vi "test_ads_surface_vapor.vi"() -> ()   [LabVIEW 2017]
doc: "Minimal example that demonstrates functions implemented in the SorpPropLib for adsorption working pairs based on the surface approach and using the vapor pressure as additional property."
panel:
  out "Der. of loading wrt. pressure":cluster{dbl[], dbl[]}[](graph)=[{[100.0, 101.0, 102.0, 103.0, 104.0, 105.0, 106.0, 107.0, 108.0, 109.0], [0.00023285248517238496, 0.0002319852444530851, 0.00023112973054732367, 0.00023028567222781486, 0.00022945280709583772, 0.00022863088121227149, 0.0002278196487473965, 0.000227018871648338, 0.00022622831932311063, 0.00022544776834028737]}, {[100.0, 101.0, 102.0, 103.0, 104.0, 105.0, 106.0, 107.0, 108.0, 109.0], [0.00023285248517238496, 0.0002319852444530851, 0.00023112973054732367, 0.00023028567222781486, 0.00022945280709583772, 0.00022863088121227149, 0.0002278196487473965, 0.000227018871648338, 0.00022622831932311063, 0.00022544776834028737]}]
  out "Der. of loading wrt. temperature":cluster{dbl[], dbl[]}[](graph)=[{[100.0, 101.0, 102.0, 103.0, 104.0, 105.0, 106.0, 107.0, 108.0, 109.0], [-0.0013688715249931432, -0.00137741100365092, -0.001385918834498026, -0.0013943954433897668, -0.0014028412463793875, -0.0014112566500356107, -0.0014196420517469718, -0.0014279978400136102, -0.001436324394727153, -0.0014446220874392785]}, {[100.0, 101.0, 102.0, 103.0, 104.0, 105.0, 106.0, 107.0, 108.0, 109.0], [-0.0013688715249931432, -0.00137741100365092, -0.001385918834498026, -0.0013943954433897668, -0.0014028412463793875, -0.0014112566500356107, -0.0014196420517469718, -0.0014279978400136102, -0.001436324394727153, -0.0014446220874392785]}]
  out "Der. of pressure wrt. loading":cluster{dbl[], dbl[]}[](graph)=[{[100.0, 101.0, 102.0, 103.0, 104.0, 105.0, 106.0, 107.0, 108.0, 109.0], [4294.5644288901685, 4310.6189893997, 4326.574507018043, 4342.43255486051, 4358.1946660705735, 4373.862335209011, 4389.437019582042, 4404.920140511679, 4420.313084551319, 4435.6172046494385]}, {[100.0, 101.0, 102.0, 103.0, 104.0, 105.0, 106.0, 107.0, 108.0, 109.0], [4294.5644288901685, 4310.6189893997, 4326.574507018043, 4342.43255486051, 4358.1946660705735, 4373.862335209011, 4389.437019582042, 4404.920140511679, 4420.313084551319, 4435.6172046494385]}]
  out "Der. of pressure wrt. temperature":cluster{dbl[], dbl[]}[](graph)=[{[100.0, 101.0, 102.0, 103.0, 104.0, 105.0, 106.0, 107.0, 108.0, 109.0], [5.878706958956192, 5.937494028545754, 5.996281098135316, 6.055068167724879, 6.11385523731444, 6.172642306904002, 6.231429376493563, 6.290216446083125, 6.349003515672687, 6.40779058526225]}, {[100.0, 101.0, 102.0, 103.0, 104.0, 105.0, 106.0, 107.0, 108.0, 109.0], [5.878706958956192, 5.937494028545754, 5.996281098135316, 6.055068167724879, 6.11385523731444, 6.172642306904002, 6.231429376493563, 6.290216446083125, 6.349003515672687, 6.40779058526225]}]
  out "Temperature":cluster{dbl[], dbl[]}[](graph)=[{[100.0, 101.0, 102.0, 103.0, 104.0, 105.0, 106.0, 107.0, 108.0, 109.0], [300.00000000000006, 300.00000000000006, 300.00000000000006, 300.00000000000006, 300.00000000000006, 300.00000000000006, 300.00000000000006, 300.00000000000006, 300.00000000000006, 300.00000000000006]}, {[100.0, 101.0, 102.0, 103.0, 104.0, 105.0, 106.0, 107.0, 108.0, 109.0], [300.00000000000006, 300.00000000000006, 300.00000000000006, 300.00000000000006, 300.00000000000006, 300.00000000000006, 300.00000000000006, 300.00000000000006, 300.00000000000006, 300.00000000000006]}]
  out "Pressure":cluster{dbl[], dbl[]}[](graph)=[{[100.0, 101.0, 102.0, 103.0, 104.0, 105.0, 106.0, 107.0, 108.0, 109.0], [99.99999999999999, 100.99999999999999, 101.99999999999999, 102.99999999999999, 103.99999999999999, 104.99999999999999, 105.99999999999996, 106.99999999999997, 107.99999999999997, 108.99999999999997]}, {[100.0, 101.0, 102.0, 103.0, 104.0, 105.0, 106.0, 107.0, 108.0, 109.0], [99.99999999999999, 100.99999999999999, 101.99999999999999, 102.99999999999999, 103.99999999999999, 104.99999999999999, 105.99999999999996, 106.99999999999997, 107.99999999999997, 108.99999999999997]}]
  out "Loading":cluster{dbl[], dbl[]}[](graph)=[{[100.0, 101.0, 102.0, 103.0, 104.0, 105.0, 106.0, 107.0, 108.0, 109.0], [0.037256397627581594, 0.03748881550361855, 0.03772037202532322, 0.03795107878314388, 0.03818094710074739, 0.038409988043661615, 0.03863821242755844, 0.038865630826195464, 0.039092253579033516, 0.03931809079854612]}, {[100.0, 101.0, 102.0, 103.0, 104.0, 105.0, 106.0, 107.0, 108.0, 109.0], [0.037256397627581594, 0.03748881550361855, 0.03772037202532322, 0.03795107878314388, 0.03818094710074739, 0.038409988043661615, 0.03863821242755844, 0.038865630826195464, 0.039092253579033516, 0.03931809079854612]}]
  in  "WorkingPair (Input)":T1={"no_iso"=1, "no_p_sat"=1, "path_db"="D:\\Driesel\\SorpLibLocal\\labview_wrapper\\data\\json\\sorpproplib.json", "wp_as"="silica gel pellet", "wp_st"="Fuji A", "wp_iso"="Freundlich", "wp_rf"="Water", "rf_rhol"="SaturatedLiquidDensity_EoS1", "no_rhol"=1, "rf_psat"="VaporPressure_EoS1"}
  in  "Temperature in K (Input)":dbl=300.0
  in  "Pressure in Pa (Input)":dbl=100.0
  # "Increase pressure by 5 Pa in steps of 1 Pa."
  # "Path to database"
  # "Name of sorbent"
  # "Name of sub-type of sorbent"
  # "Name of refrigerant"
  # "Name of isotherm"
  # "ID of isotherm"
  # "Name of calculation approach for vapor pressure"
  # "ID of vapor pressure equation"
  # "Name of calculation approach for liquid density"
  # "ID of liquid density equation"
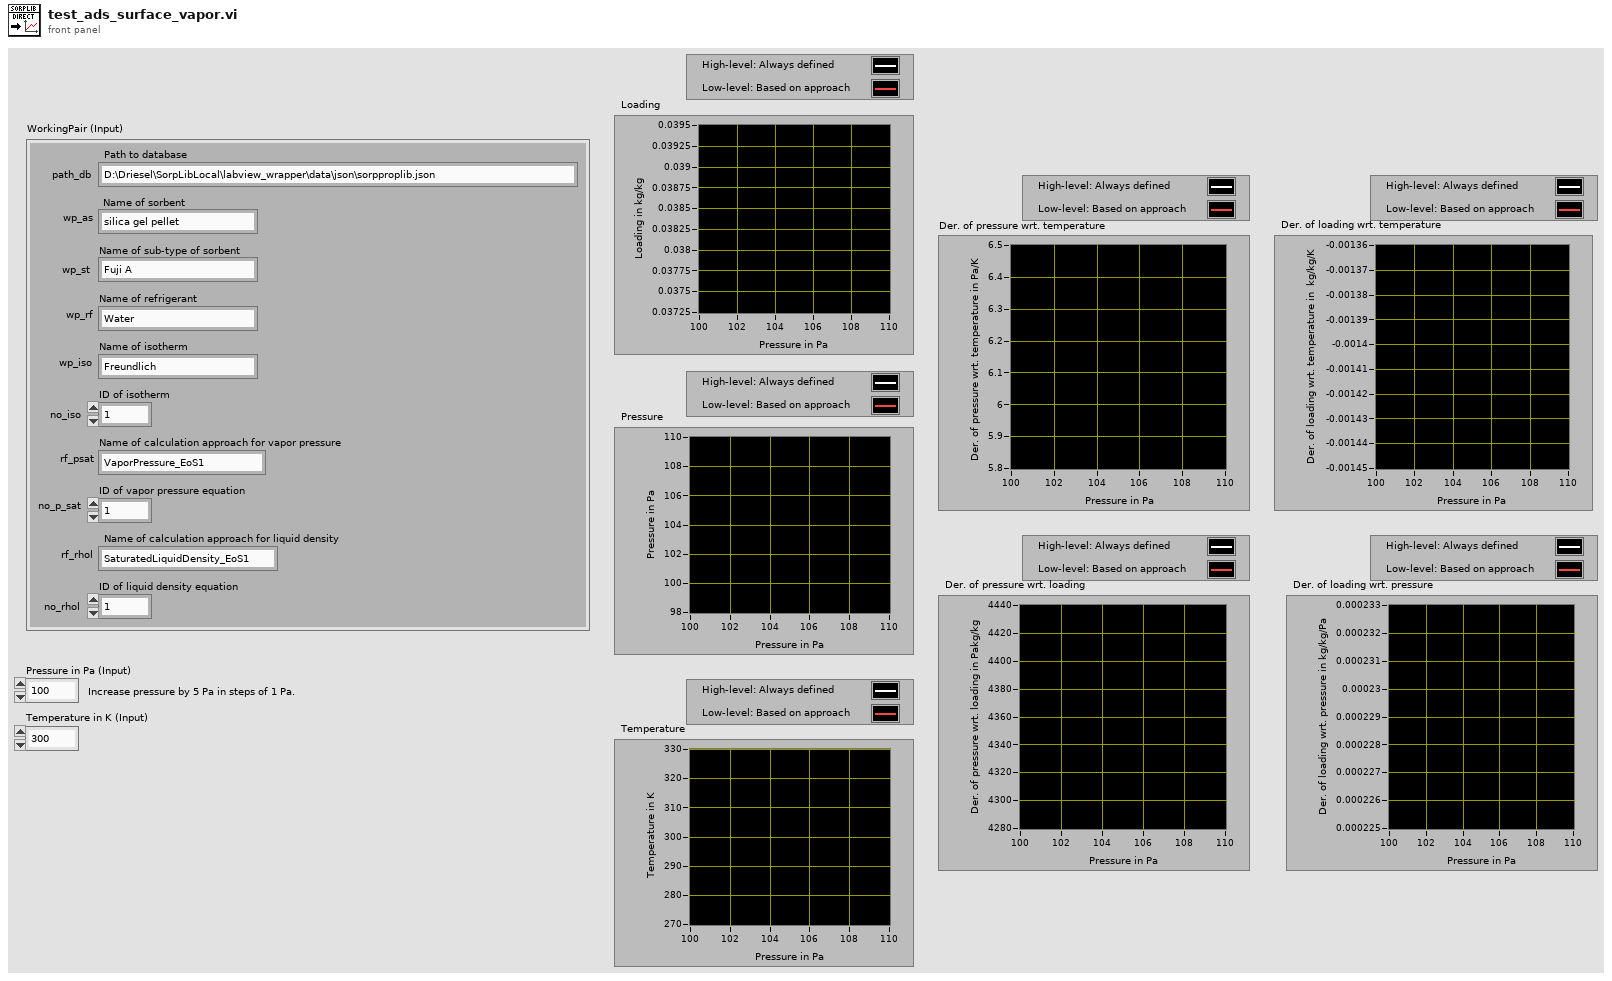
[diagram p1: front panel]
types:
  T1 = cluster{"no_iso":i32, "no_p_sat":i32, "path_db":string, "wp_as":string, "wp_st":string, "wp_iso":string, "wp_rf":string, "rf_rhol":string, "no_rhol":i32, "rf_psat":string}
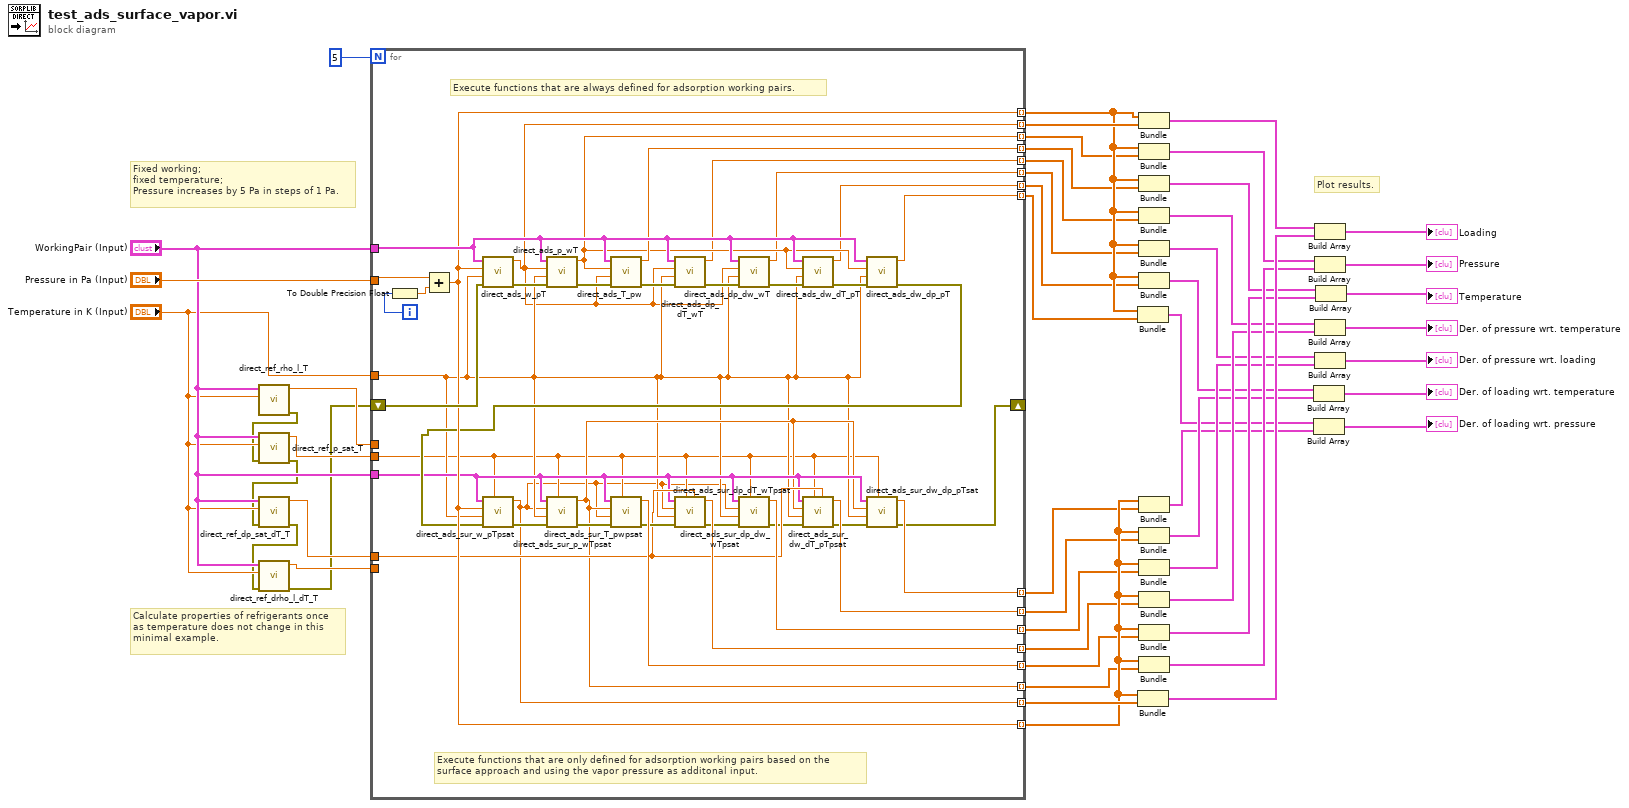
[diagram p0: block diagram]
diagram:
  # "Fixed working;\nfixed temperature;\nPressure increases by 5 Pa in steps of 1 Pa."
  # "Plot results."
  # "Calculate properties of refrigerants once\nas temperature does not change in this\nminimal example."
  n1 = call "direct_ref_rho_l_T.vi"("Temperature in K (Input)"="Temperature in K (Input)", "WorkingPair (Input)"="WorkingPair (Input)") -> ("Error (Output)"=w4:errorcluster, "Saturated liquid density in kg/m3 (Output)"=w8:dbl)  [unwired: 8 in]
  n2 = call "direct_ref_p_sat_T.vi"("Error (Input)"=w4, "Temperature in K (Input)"="Temperature in K (Input)", "WorkingPair (Input)"="WorkingPair (Input)") -> ("Error (Output)"=w3:errorcluster, "Saturation pressure in Pa (Output)"=w5:dbl)  [unwired: 7 in]
  n3 = call "direct_ref_dp_sat_dT_T.vi"("Error (Input)"=w3, "Temperature in K (Input)"="Temperature in K (Input)", "WorkingPair (Input)"="WorkingPair (Input)") -> ("Error (Output)"=w2:errorcluster, "Der. of saturation pressure wrt temperature in Pa/K (Output)"=w10:dbl)  [unwired: 7 in]
  n4 = call "direct_ref_drho_l_dT_T.vi"("Error (Input)"=w2, "Temperature in K (Input)"="Temperature in K (Input)", "WorkingPair (Input)"="WorkingPair (Input)") -> ("Error (Output)"=w1:errorcluster, "Der. of saturated liquid density wrt temperature in kg/m3/K (Output)"=w9:dbl)  [unwired: 7 in]
  n5 = for {
    N: 5 -> [_]
    tunnel: "Pressure in Pa (Input)" -> [w87]
    tunnel: "Temperature in K (Input)" -> [w56]
    tunnel: "WorkingPair (Input)" -> [w82]
    shift-right: [w50] -> _
    shift-left: w1 -> [w71]
    tunnel: [w77] -> w44 mode=indexing
    tunnel: [w70] -> w46 mode=indexing
    tunnel: [w52] -> w47 mode=indexing
    tunnel: [w76] -> w45 mode=indexing
    tunnel: [w75] -> w43 mode=indexing
    tunnel: [w74] -> w42 mode=indexing
    tunnel: [w73] -> w40 mode=indexing
    tunnel: [w72] -> w41 mode=indexing
    tunnel: "WorkingPair (Input)" -> [w58]
    tunnel: w5 -> [w53]
    tunnel: w8 -> [_]
    tunnel: [w51] -> w39 mode=indexing
    tunnel: [w70] -> w38 mode=indexing
    tunnel: [w57] -> w37 mode=indexing
    tunnel: [w66] -> w36 mode=indexing
    tunnel: [w64] -> w25 mode=indexing
    tunnel: [w62] -> w22 mode=indexing
    tunnel: [w59] -> w18 mode=indexing
    tunnel: [w55] -> w17 mode=indexing
    tunnel: w10 -> [w61]
    tunnel: w9 -> [_]
    i -> [w86]
    # "Execute functions that are only defined for adsorption working pairs based on the\nsurface approach and using the vapor pressure as additonal input."
    # "Execute functions that are always defined for adsorption working pairs."
    n6 = To Double Precision Float(number=w86) -> (double precision float=w85:dbl)
    n7 = Add(x=w87, y=w85) -> (x+y=w70:dbl)
    n8 = call "direct_ads_w_pT.vi"("Error (Input)"=w71, "Temperature in K (Input)"=w56, "Pressure in Pa (Input)"=w70, "WorkingPair (Input)"=w82) -> ("Error (Output)"=w84:errorcluster, "Loading in kg/kg (Output)"=w52:dbl)  [unwired: 6 in]
    n9 = call "direct_ads_p_wT.vi"("Error (Input)"=w84, "Temperature in K (Input)"=w56, "Loading in kg/kg (Input)"=w52, "WorkingPair (Input)"=w82) -> ("Error (Output)"=w83:errorcluster, "Pressure in Pa (Output)"=w76:dbl)  [unwired: 6 in]
    n10 = call "direct_ads_T_pw.vi"("Error (Input)"=w83, "Loading in kg/kg (Input)"=w52, "Pressure in Pa (Input)"=w76, "WorkingPair (Input)"=w82) -> ("Error (Output)"=w81:errorcluster, "Temperature in K (Output)"=w77:dbl)  [unwired: 6 in]
    n11 = call "direct_ads_dp_dT_wT.vi"("Error (Input)"=w81, "Temperature in K (Input)"=w56, "Loading in kg/kg (Input)"=w52, "WorkingPair (Input)"=w82) -> ("Error (Output)"=w80:errorcluster, "Der. of pressure wrt. temperature in Pa/K (Output)"=w75:dbl)  [unwired: 6 in]
    n12 = call "direct_ads_dp_dw_wT.vi"("Error (Input)"=w80, "Temperature in K (Input)"=w56, "Loading in kg/kg (Input)"=w52, "WorkingPair (Input)"=w82) -> ("Error (Output)"=w79:errorcluster, "Der. of pressure wrt. loading in Pakg/kg (Output)"=w74:dbl)  [unwired: 6 in]
    n13 = call "direct_ads_dw_dT_pT.vi"("Error (Input)"=w79, "Temperature in K (Input)"=w56, "Pressure in Pa (Input)"=w76, "WorkingPair (Input)"=w82) -> ("Error (Output)"=w78:errorcluster, "Der. of loading wrt. temperature in kg/kg/K (Output)"=w73:dbl)  [unwired: 6 in]
    n14 = call "direct_ads_dw_dp_pT.vi"("Error (Input)"=w78, "Temperature in K (Input)"=w56, "Pressure in Pa (Input)"=w76, "WorkingPair (Input)"=w82) -> ("Error (Output)"=w69:errorcluster, "Der. of loading wrt. pressure in kg/kg/Pa (Output)"=w72:dbl)  [unwired: 6 in]
    n15 = call "direct_ads_sur_w_pTpsat.vi"("Saturation vapor pressure in Pa (Input)"=w53, "Error (Input)"=w69, "Temperature in K (Input)"=w56, "Pressure in Pa (Input)"=w70, "WorkingPair (Input)"=w58) -> ("Error (Output)"=w68:errorcluster, "Equilibrium loading in kg/kg (Output)"=w51:dbl)  [unwired: 5 in]
    n16 = call "direct_ads_sur_p_wTpsat.vi"("Saturation vapor pressure in Pa (Input)"=w53, "Error (Input)"=w68, "Temperature in K (Input)"=w56, "Loading in kg/kg (Input)"=w51, "WorkingPair (Input)"=w58) -> ("Error (Output)"=w67:errorcluster, "Equilibrium pressure in Pa (Output)"=w57:dbl)  [unwired: 5 in]
    n17 = call "direct_ads_sur_T_pwpsat.vi"("Saturation vapor pressure in Pa (Input)"=w53, "Error (Input)"=w67, "Loading in kg/kg (Input)"=w51, "Pressure in Pa (Input)"=w57, "WorkingPair (Input)"=w58) -> ("Error (Output)"=w65:errorcluster, "Equilibrium temperature in K (Output)"=w66:dbl)  [unwired: 5 in]
    n18 = call "direct_ads_sur_dp_dT_wTpsat.vi"("Der. of saturation pressure wrt. temperature in Pa/K (Input)"=w61, "Saturation vapor pressure in Pa (Input)"=w53, "Error (Input)"=w65, "Temperature in K (Input)"=w56, "Loading in kg/kg (Input)"=w51, "WorkingPair (Input)"=w58) -> ("Error (Output)"=w63:errorcluster, "Der. pressure wrt. temperature in Pa/K (Output)"=w64:dbl)  [unwired: 4 in]
    n19 = call "direct_ads_sur_dp_dw_wTpsat.vi"("Saturation vapor pressure in Pa (Input)"=w53, "Error (Input)"=w63, "Temperature in K (Input)"=w56, "Loading in kg/kg (Input)"=w51, "WorkingPair (Input)"=w58) -> ("Error (Output)"=w60:errorcluster, "Der. pressure wrt. loading in Pakg/kg (Output)"=w62:dbl)  [unwired: 5 in]
    n20 = call "direct_ads_sur_dw_dT_pTpsat.vi"("Der. of saturation pressure wrt. temperature in Pa/K (Input)"=w61, "Saturation vapor pressure in Pa (Input)"=w53, "Error (Input)"=w60, "Temperature in K (Input)"=w56, "Pressure in Pa (Input)"=w57, "WorkingPair (Input)"=w58) -> ("Error (Output)"=w54:errorcluster, "Der. loading wrt. tempreature in kg/kg/K (Output)"=w59:dbl)  [unwired: 4 in]
    n21 = call "direct_ads_sur_dw_dp_pTsat.vi"("Saturation vapor pressure in Pa (Input)"=w53, "Error (Input)"=w54, "Temperature in K (Input)"=w56, "Pressure in Pa (Input)"=w57, "WorkingPair (Input)"=w58) -> ("Error (Output)"=w50:errorcluster, "Der. of loading wrt. pressure in kg/kg/Pa (Output)"=w55:dbl)  [unwired: 5 in]
  }
  n22 = Bundle(w46, w41) -> (w14:cluster{dbl[], dbl[]})  [unwired: 1 in]
  n23 = Bundle(w38, w39) -> (w34:cluster{dbl[], dbl[]})  [unwired: 1 in]
  n24 = Bundle(w46, w47) -> (w35:cluster{dbl[], dbl[]})  [unwired: 1 in]
  n25 = Bundle(w46, w45) -> (w33:cluster{dbl[], dbl[]})  [unwired: 1 in]
  n26 = Bundle(w46, w44) -> (w31:cluster{dbl[], dbl[]})  [unwired: 1 in]
  n27 = Bundle(w46, w43) -> (w29:cluster{dbl[], dbl[]})  [unwired: 1 in]
  n28 = Bundle(w46, w42) -> (w21:cluster{dbl[], dbl[]})  [unwired: 1 in]
  n29 = Bundle(w46, w40) -> (w16:cluster{dbl[], dbl[]})  [unwired: 1 in]
  n30 = Bundle(w38, w17) -> (w13:cluster{dbl[], dbl[]})  [unwired: 1 in]
  n31 = Bundle(w38, w18) -> (w15:cluster{dbl[], dbl[]})  [unwired: 1 in]
  n32 = Bundle(w38, w22) -> (w20:cluster{dbl[], dbl[]})  [unwired: 1 in]
  n33 = Bundle(w38, w25) -> (w24:cluster{dbl[], dbl[]})  [unwired: 1 in]
  n34 = Bundle(w38, w36) -> (w30:cluster{dbl[], dbl[]})  [unwired: 1 in]
  n35 = Bundle(w38, w37) -> (w32:cluster{dbl[], dbl[]})  [unwired: 1 in]
  n36 = Build Array(w16, w15) -> (→"Der. of loading wrt. temperature":cluster{dbl[], dbl[]}[])
  n37 = Build Array(w14, w13) -> (→"Der. of loading wrt. pressure":cluster{dbl[], dbl[]}[])
  n38 = Build Array(w35, w34) -> (→"Loading":cluster{dbl[], dbl[]}[])
  n39 = Build Array(w33, w32) -> (→"Pressure":cluster{dbl[], dbl[]}[])
  n40 = Build Array(w29, w24) -> (→"Der. of pressure wrt. temperature":cluster{dbl[], dbl[]}[])
  n41 = Build Array(w21, w20) -> (→"Der. of pressure wrt. loading":cluster{dbl[], dbl[]}[])
  n42 = Build Array(w31, w30) -> (→"Temperature":cluster{dbl[], dbl[]}[])
